vi "Command Arm.vi"(7 "Startup":bool, 9 "Timeout":u32, 10 "Set Position":T1=enum."Climb") -> (3 "Arm Out":dbl, 4 "Reinit":bool, 6 "Completed":bool)   [LabVIEW 2017]
uses:
  Intake Rotation/Arm Enum States.ctl
  Intake Rotation/Intake Rotation Globals.vi
  Lift/Lift Globals.vi
panel:
  out "Maintain Position":i32
  in  "Lift Point":i32=6000
  in  "Kp Up":dbl=0.0003
  in  "Kp Down":dbl=0.0003
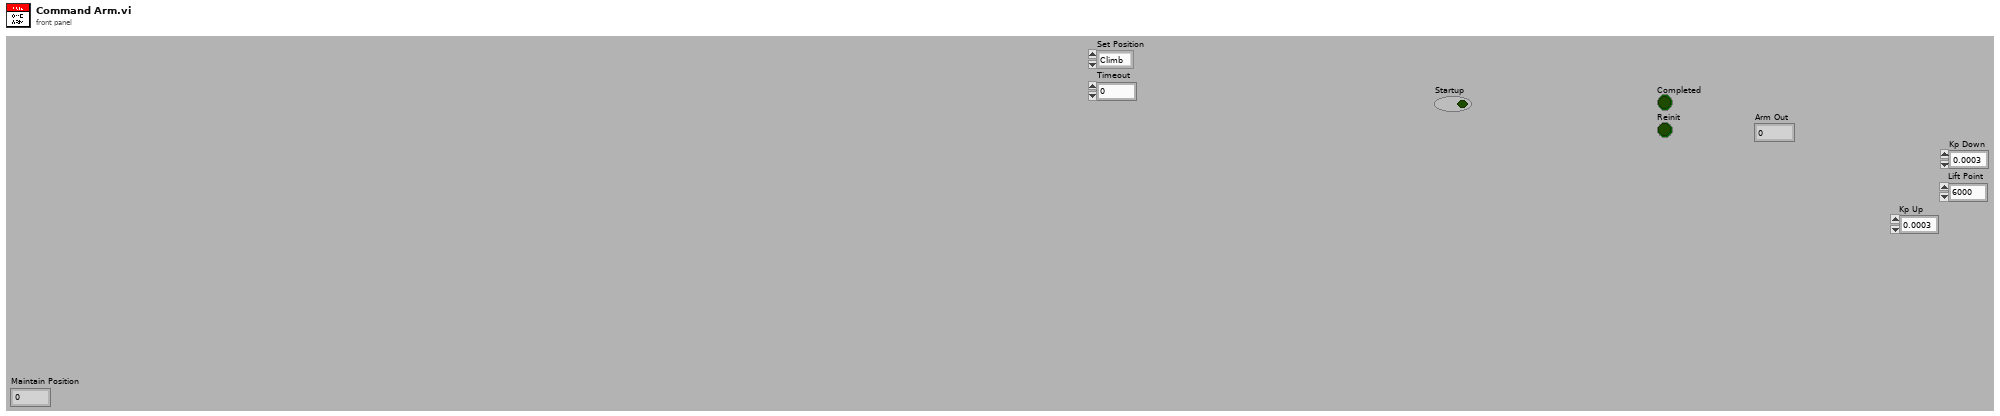
[diagram p1: front panel]
types:
  T1 = typedef "Arm Enum States.ctl" = enum16{"Current Position", "Climb", "Load", "Portal", "Switch", "Scale High", "Scale Mid", "Scale Low", "Exchange", "Stow"}
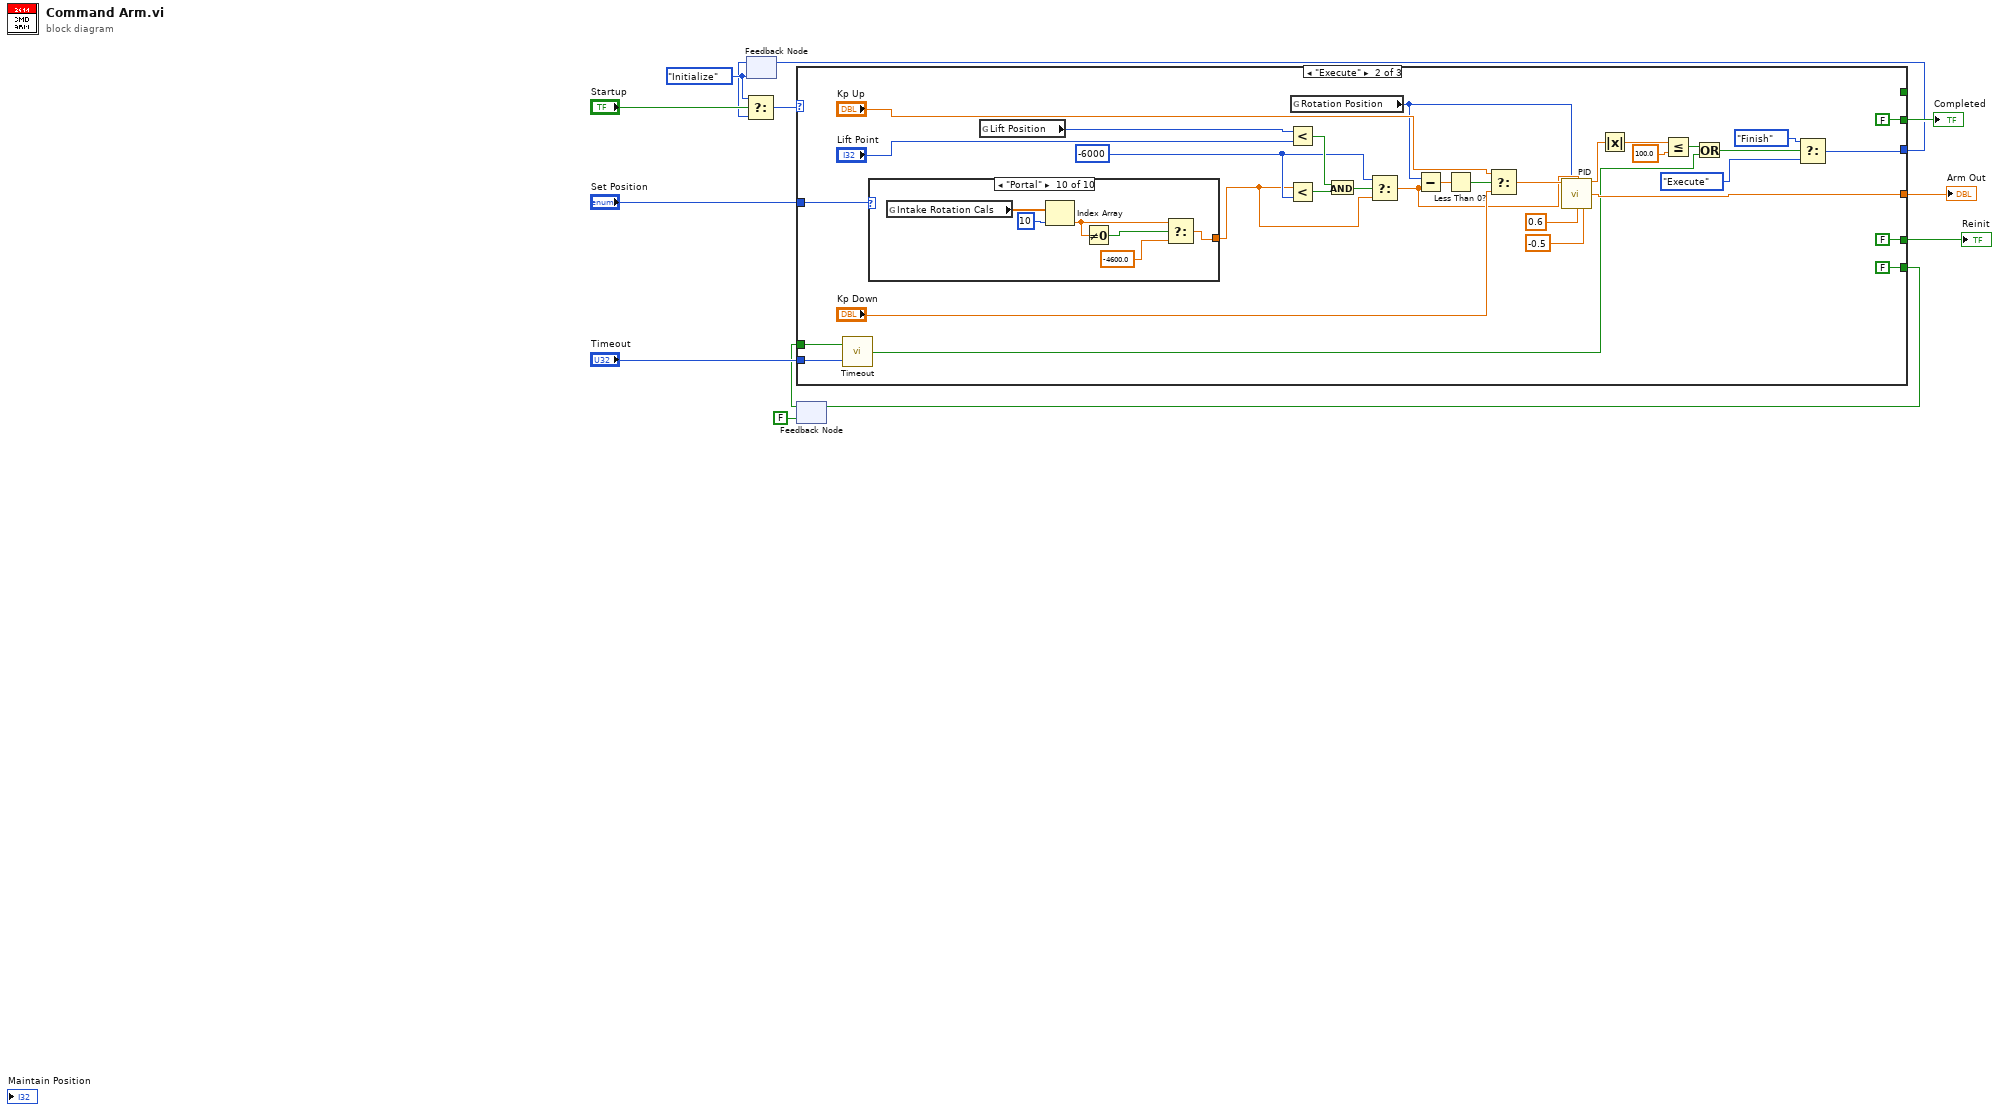
[diagram p0: block diagram]
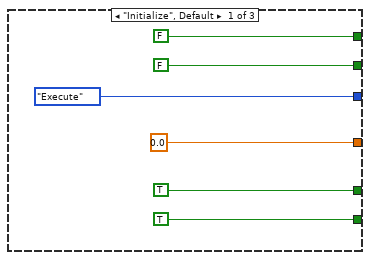
[diagram p2: hidden frame]
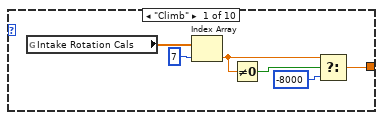
[diagram p3: hidden frame]
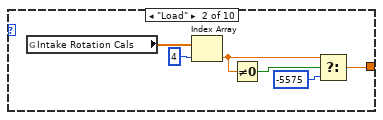
[diagram p4: hidden frame]
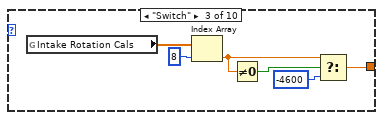
[diagram p5: hidden frame]
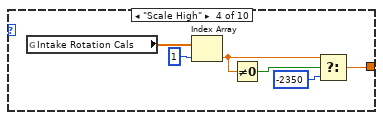
[diagram p6: hidden frame]
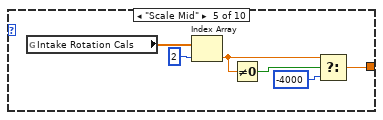
[diagram p7: hidden frame]
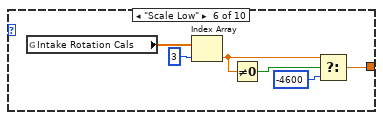
[diagram p8: hidden frame]
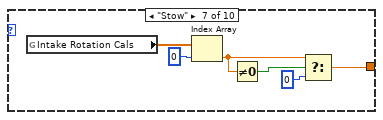
[diagram p9: hidden frame]
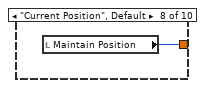
[diagram p10: hidden frame]
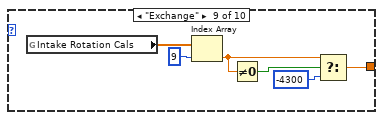
[diagram p11: hidden frame]
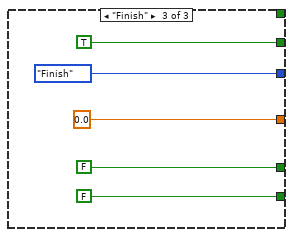
[diagram p12: hidden frame]
diagram:
  w11 = enum16{"Initialize", "Execute", "Finish"}."Initialize"
  n1 = feedback #1(w11) -> (w7:enum16{"Initialize", "Execute", "Finish"})
  n2 = Select(t=w11, s="Startup", f=w7) -> (s? t:f=w12:enum16{"Initialize", "Execute", "Finish"})
  n3 = feedback #2(FALSE) -> (w2:bool)
  n4 = case shown="\"Execute\"" w12 {
    tunnel: [FALSE FALSE TRUE] -> w10
    tunnel: [TRUE FALSE FALSE] -> w9
    tunnel: [enum16{"Initialize", "Execute", "Finish"}."Execute" w47 enum16{"Initialize", "Execute", "Finish"}."Finish"] -> w8
    tunnel: [0.0 ("Right Wheel Velocity") w46 0.0] -> w6
    tunnel: "Set Position" -> [_ w21 _]
    tunnel: [FALSE _ _] -> _
    tunnel: "Timeout" -> [_ w28 _]
    tunnel: w2 -> [_ w27 _]
    tunnel: [TRUE FALSE FALSE] -> w3
    frame "Initialize", Default {
    }
    frame "Execute" {
      w35 = -6000 ("y")
      n5 = call "Timeout.vi"("Timeout"=w28, "Initialize"=w27) -> ("Timed Out?"=w29:bool)
      n6 = case shown="\"Portal\"" w21 {
        tunnel: [w53 w58 w64 w70 w76 w82 w88 w94 w97 w101] -> w20
        frame "Climb" {
          n7 = global read "Intake Rotation Globals.vi" "Intake Rotation Cals"() -> (w57:dbl[])
          n8 = Index Array(array=w57, index=7) -> (element=w52:dbl)
          n9 = Not Equal To 0?(x=w52) -> (x != 0?=w55:bool)
          n10 = Select(t=w52, s=w55, f=-8000) -> (s? t:f=w53:dbl)
        }
        frame "Load" {
          n11 = global read "Intake Rotation Globals.vi" "Intake Rotation Cals"() -> (w63:dbl[])
          n12 = Index Array(array=w63, index=4) -> (element=w59:dbl)
          n13 = Not Equal To 0?(x=w59) -> (x != 0?=w61:bool)
          n14 = Select(t=w59, s=w61, f=-5575) -> (s? t:f=w58:dbl)
        }
        frame "Switch" {
          n15 = global read "Intake Rotation Globals.vi" "Intake Rotation Cals"() -> (w69:dbl[])
          n16 = Index Array(array=w69, index=8) -> (element=w65:dbl)
          n17 = Not Equal To 0?(x=w65) -> (x != 0?=w67:bool)
          n18 = Select(t=w65, s=w67, f=-4600) -> (s? t:f=w64:dbl)
        }
        frame "Scale High" {
          n19 = global read "Intake Rotation Globals.vi" "Intake Rotation Cals"() -> (w75:dbl[])
          n20 = Index Array(array=w75, index=1) -> (element=w71:dbl)
          n21 = Not Equal To 0?(x=w71) -> (x != 0?=w73:bool)
          n22 = Select(t=w71, s=w73, f=-2350) -> (s? t:f=w70:dbl)
        }
        frame "Scale Mid" {
          n23 = global read "Intake Rotation Globals.vi" "Intake Rotation Cals"() -> (w81:dbl[])
          n24 = Index Array(array=w81, index=2) -> (element=w77:dbl)
          n25 = Not Equal To 0?(x=w77) -> (x != 0?=w79:bool)
          n26 = Select(t=w77, s=w79, f=-4000) -> (s? t:f=w76:dbl)
        }
        frame "Scale Low" {
          n27 = global read "Intake Rotation Globals.vi" "Intake Rotation Cals"() -> (w87:dbl[])
          n28 = Index Array(array=w87, index=3) -> (element=w83:dbl)
          n29 = Not Equal To 0?(x=w83) -> (x != 0?=w85:bool)
          n30 = Select(t=w83, s=w85, f=-4600) -> (s? t:f=w82:dbl)
        }
        frame "Stow" {
          n31 = global read "Intake Rotation Globals.vi" "Intake Rotation Cals"() -> (w93:dbl[])
          n32 = Index Array(array=w93, index=0) -> (element=w89:dbl)
          n33 = Not Equal To 0?(x=w89) -> (x != 0?=w91:bool)
          n34 = Select(t=w89, s=w91, f=0) -> (s? t:f=w88:dbl)
        }
        frame "Current Position", Default {
          n35 = local read "Maintain Position"() -> (w94:i32)
        }
        frame "Exchange" {
          n36 = global read "Intake Rotation Globals.vi" "Intake Rotation Cals"() -> (w100:dbl[])
          n37 = Index Array(array=w100, index=9) -> (element=w95:dbl)
          n38 = Not Equal To 0?(x=w95) -> (x != 0?=w98:bool)
          n39 = Select(t=w95, s=w98, f=-4300) -> (s? t:f=w97:dbl)
        }
        frame "Portal" {
          n40 = global read "Intake Rotation Globals.vi" "Intake Rotation Cals"() -> (w106:dbl[])
          n41 = Index Array(array=w106, index=10) -> (element=w103:dbl)
          n42 = Not Equal To 0?(x=w103) -> (x != 0?=w104:bool)
          n43 = Select(t=w103, s=w104, f=-4600.0 ("Numeric")) -> (s? t:f=w101:dbl)
        }
      }
      n44 = global read "Lift Globals.vi" "Lift Position"() -> (w40:i32)
      n45 = Less?(x=w40, y="Lift Point") -> (x < y?=w38:bool)
      n46 = Less?(x=w20, y=w35) -> (x < y?=w37:bool)
      n47 = global read "Intake Rotation Globals.vi" "Rotation Position"() -> (w22:i32)
      n48 = And(x=w38, y=w37) -> (x .and. y?=w36:bool)
      n49 = Select(t=w35, s=w36, f=w20) -> (s? t:f=w23:dbl)
      n50 = Subtract(x=w22, y=w23) -> (x-y=w45:dbl)
      n51 = Less Than 0?(x=w45) -> (x < 0?=w44:bool)
      n52 = Select(t="Kp Up", s=w44, f="Kp Down") -> (s? t:f=w43:dbl)
      n53 = call "PID.vi"("Kp"=w43, "Process Variable"=w22, "Goal"=w23, "Max Ouput"=0.6, "Min Output"=-0.5) -> ("Current Error"=w34:dbl, "Command"=w46:dbl)  [unwired: 8 in, 1 out]
      n54 = Absolute Value(x=w34) -> (abs(x)=w32:dbl)
      n55 = Less Or Equal?(x=w32, y=100.0) -> (x <= y?=w31:bool)
      n56 = Or(x=w31, y=w29) -> (x .or. y?=w30:bool)
      n57 = Select(t=enum16{"Initialize", "Execute", "Finish"}."Finish", s=w30, f=enum16{"Initialize", "Execute", "Finish"}."Execute") -> (s? t:f=w47:enum16{"Initialize", "Execute", "Finish"})
    }
    frame "Finish" {
    }
  }
  "Completed" <- w10
  "Reinit" <- w9
  "Arm Out" <- w6
  n58 = feedback-in #1(w8) -> ()
  n59 = feedback-in #2(w3) -> ()
